vi "LabVIEW_INI_FIX_Fonts_2011.vi"() -> ()   [LabVIEW 2011]
uses:
  <vilib>/registry/registry.llb/Registry RtKey.ctl
  <vilib>/registry/registry.llb/Registry SAM.ctl
  <vilib>/Utility/config.llb/Read Key (String).vi
  <vilib>/Utility/config.llb/Write Key (String).vi
  <vilib>/Utility/config.llb/NI_LVConfig.lvlib
panel:
  out "total fonts info in registry":T1
  out "all fonts array":string[](array[string])
  out "Fonts sorted":string[](array[string])
  out "previous value in ini":string
  out "Fonts value to write in ini":string
  out "All found labVIEW.INI in Default Dir":path[](array[path])
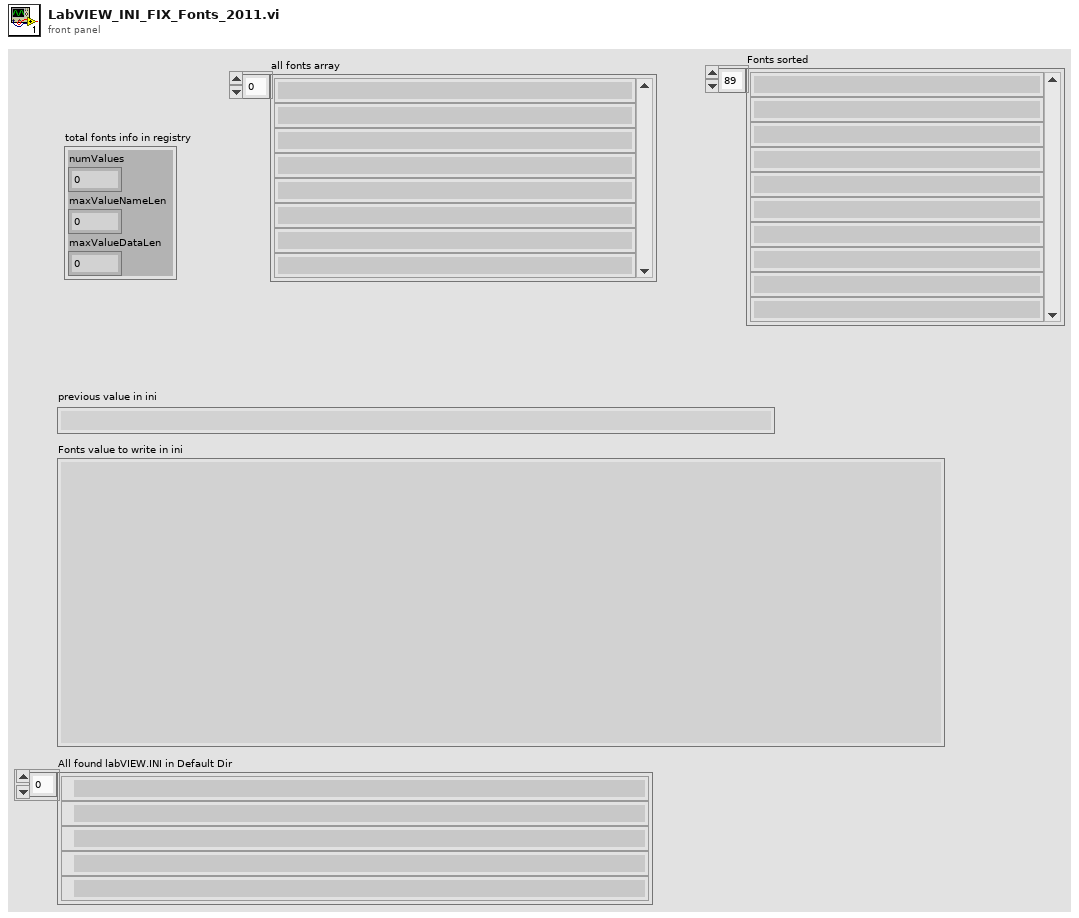
[diagram p1: front panel]
types:
  T1 = cluster{"numValues":i32, "maxValueNameLen":i32, "maxValueDataLen":i32}
  T2 = typedef "Registry SAM.ctl" = enum32{"KEY_QUERY_VALUE", "KEY_SET_VALUE", "KEY_CREATE_SUB_KEY", "KEY_ENUMERATE_SUB_KEYS", "KEY_NOTIFY", "KEY_CREATE_LINK", "KEY_READ", "KEY_WRITE", "KEY_ALL_ACCESS", "KEY_READ | KEY_WRITE"}
  T3 = typedef "Registry RtKey.ctl" = enum32{"HKEY_CLASSES_ROOT", "HKEY_CURRENT_USER", "HKEY_LOCAL_MACHINE", "HKEY_USERS", "HKEY_PERFORMANCE_DATA", "HKEY_CURRENT_CONFIG", "HKEY_DYN_DATA"}
  T4 = typedef "Registry refnum.ctl" = refnum<k1>
  T5 = typedef "NI_LVConfig.lvlib/Config Data RefNum.ctl" = refnum<k1>
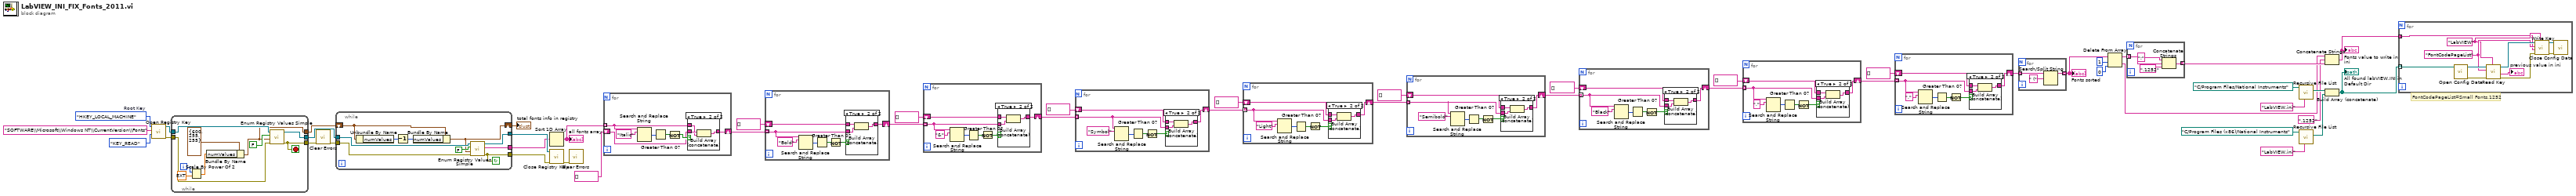
[diagram p0: block diagram]
diagram:
  w34 = Registry_RtKey."HKEY_LOCAL_MACHINE"  # Root Key
  # "FontCodePageList=Small Fonts,1252"
  n1 = call <vilib>:"Open Registry Key.vi"("security access mask (KEY_READ | KEY_WRITE)"=Registry_SAM."KEY_READ", "subkey"="SOFTWARE\\Microsoft\\Windows NT\\CurrentVersion\\Fonts", "root key (HKEY_LOCAL_MACHINE)"=w34) -> ("error out"=w15:errorcluster, "refnum out"=w18:T4)  [unwired: 7 in]
  n2 = while {
    tunnel: w18 -> [w57]
    tunnel: [w55] -> w19
    tunnel: [w51] -> w20
    tunnel: w15 -> [w50]
    tunnel: [w49] -> w14
    i -> [w54]
    stop <- w49 stop-if-true
    n3 = Scale By Power Of 2(n=w54, x=ext 1.0) -> (x*2^n=w52:ext)
    n4 = Bundle By Name(cluster=T1 {"numValues"=600, "maxValueNameLen"=255, "maxValueDataLen"=255} ("value info"), "numValues"=w52) -> (w51:T1)
    n5 = call <vilib>:"Enum Registry Values Simple.vi"("error in (no error)"=w50, "value info"=w51, "retrieve data? (F)"=FALSE, "refnum"=w57) -> ("error out"=w49:errorcluster, "refnum out"=w55:T4)  [unwired: 2 in, 4 out]
  }
  n6 = call <vilib>:"Clear Errors.vi"("error in (no error)"=w14) -> ("error out"=w12:errorcluster)  [unwired: 6 in]
  n7 = while {
    shift-right: [w62] -> w11
    shift-left: w20 -> [w67]
    tunnel: w19 -> [w64]
    tunnel: [w63] -> w17
    tunnel: [w61] -> w16
    tunnel: w12 -> [w60]
    tunnel: [w59] -> w13
    stop <- w59 continue-if-true
    n8 = Unbundle By Name(w67) -> ("numValues"=w66:i32)
    n9 = Decrement(x=w66) -> (x-1=w65:i32)
    n10 = Bundle By Name(cluster=w67, "numValues"=w65) -> (w62:T1)
    n11 = call <vilib>:"Enum Registry Values Simple.vi"("error in (no error)"=w60, "value info"=w62, "retrieve data? (F)"=FALSE, "refnum"=w64) -> ("error out"=w59:errorcluster, "values"=w61:string[], "refnum out"=w63:T4)  [unwired: 2 in, 3 out]
  }
  "total fonts info in registry" <- w11
  n12 = Sort 1D Array(array=w16) -> (sorted array=w26:string[])
  "all fonts array" <- w26
  n13 = call <vilib>:"Close Registry Key.vi"("error in (no error)"=w13, "refnum"=w17) -> ("error out"=w21:errorcluster)  [unwired: 5 in]
  n14 = call <vilib>:"Clear Errors.vi"("error in (no error)"=w21) -> ()  [unwired: 6 in, 1 out]
  n15 = for {
    tunnel: w26 -> [w72] mode=indexing
    shift-right: [w69] -> w31
    shift-left: string[] [] ("Array") -> [w70]
    n16 = Search and Replace String(input string=w72, search string="Italic") -> (number of replacements=w74:i32)  [unwired: 6 in, 3 out]
    n17 = Greater Than 0?(x=w74) -> (x > 0?=w73:bool)
    n18 = Not(x=w73) -> (.not. x?=w71:bool)
    n19 = case shown="True" w71 {
      tunnel: w70 -> [w76 w78]
      tunnel: w72 -> [_ w77]
      tunnel: [w76 w79] -> w69
      frame False {
      }
      frame True {
        n20 = Build Array (concatenate)(w78, w77) -> (w79:string[])
      }
    }
  }
  n21 = for {
    tunnel: w31 -> [w83] mode=indexing
    shift-right: [w80] -> w30
    shift-left: string[] [] ("Array") -> [w81]
    n22 = Search and Replace String(input string=w83, search string="Bold") -> (number of replacements=w85:i32)  [unwired: 6 in, 3 out]
    n23 = Greater Than 0?(x=w85) -> (x > 0?=w84:bool)
    n24 = Not(x=w84) -> (.not. x?=w82:bool)
    n25 = case shown="True" w82 {
      tunnel: w81 -> [w87 w89]
      tunnel: w83 -> [_ w88]
      tunnel: [w87 w90] -> w80
      frame False {
      }
      frame True {
        n26 = Build Array (concatenate)(w89, w88) -> (w90:string[])
      }
    }
  }
  n27 = for {
    tunnel: w30 -> [w94] mode=indexing
    shift-right: [w91] -> w29
    shift-left: string[] [] ("Array") -> [w92]
    n28 = Search and Replace String(input string=w94, search string="&") -> (number of replacements=w96:i32)  [unwired: 6 in, 3 out]
    n29 = Greater Than 0?(x=w96) -> (x > 0?=w95:bool)
    n30 = Not(x=w95) -> (.not. x?=w93:bool)
    n31 = case shown="True" w93 {
      tunnel: w92 -> [w98 w100]
      tunnel: w94 -> [_ w99]
      tunnel: [w98 w101] -> w91
      frame False {
      }
      frame True {
        n32 = Build Array (concatenate)(w100, w99) -> (w101:string[])
      }
    }
  }
  n33 = for {
    tunnel: w29 -> [w105] mode=indexing
    shift-right: [w102] -> w28
    shift-left: string[] [] ("Array") -> [w103]
    n34 = Search and Replace String(input string=w105, search string="Symbol") -> (number of replacements=w107:i32)  [unwired: 6 in, 3 out]
    n35 = Greater Than 0?(x=w107) -> (x > 0?=w106:bool)
    n36 = Not(x=w106) -> (.not. x?=w104:bool)
    n37 = case shown="True" w104 {
      tunnel: w103 -> [w109 w111]
      tunnel: w105 -> [_ w110]
      tunnel: [w109 w112] -> w102
      frame False {
      }
      frame True {
        n38 = Build Array (concatenate)(w111, w110) -> (w112:string[])
      }
    }
  }
  n39 = for {
    tunnel: w28 -> [w116] mode=indexing
    shift-right: [w113] -> w27
    shift-left: string[] [] ("Array") -> [w114]
    n40 = Search and Replace String(input string=w116, search string="Light") -> (number of replacements=w118:i32)  [unwired: 6 in, 3 out]
    n41 = Greater Than 0?(x=w118) -> (x > 0?=w117:bool)
    n42 = Not(x=w117) -> (.not. x?=w115:bool)
    n43 = case shown="True" w115 {
      tunnel: w114 -> [w120 w122]
      tunnel: w116 -> [_ w121]
      tunnel: [w120 w123] -> w113
      frame False {
      }
      frame True {
        n44 = Build Array (concatenate)(w122, w121) -> (w123:string[])
      }
    }
  }
  n45 = for {
    tunnel: w27 -> [w127] mode=indexing
    shift-right: [w124] -> w25
    shift-left: string[] [] ("Array") -> [w125]
    n46 = Search and Replace String(input string=w127, search string="Semibold") -> (number of replacements=w129:i32)  [unwired: 6 in, 3 out]
    n47 = Greater Than 0?(x=w129) -> (x > 0?=w128:bool)
    n48 = Not(x=w128) -> (.not. x?=w126:bool)
    n49 = case shown="True" w126 {
      tunnel: w125 -> [w131 w133]
      tunnel: w127 -> [_ w132]
      tunnel: [w131 w134] -> w124
      frame False {
      }
      frame True {
        n50 = Build Array (concatenate)(w133, w132) -> (w134:string[])
      }
    }
  }
  n51 = for {
    tunnel: w25 -> [w138] mode=indexing
    shift-right: [w135] -> w24
    shift-left: string[] [] ("Array") -> [w136]
    n52 = Search and Replace String(input string=w138, search string="Black") -> (number of replacements=w140:i32)  [unwired: 6 in, 3 out]
    n53 = Greater Than 0?(x=w140) -> (x > 0?=w139:bool)
    n54 = Not(x=w139) -> (.not. x?=w137:bool)
    n55 = case shown="True" w137 {
      tunnel: w136 -> [w142 w144]
      tunnel: w138 -> [_ w143]
      tunnel: [w142 w145] -> w135
      frame False {
      }
      frame True {
        n56 = Build Array (concatenate)(w144, w143) -> (w145:string[])
      }
    }
  }
  n57 = for {
    tunnel: w24 -> [w149] mode=indexing
    shift-right: [w146] -> w23
    shift-left: string[] [] ("Array") -> [w147]
    n58 = Search and Replace String(input string=w149, search string=",") -> (number of replacements=w151:i32)  [unwired: 6 in, 3 out]
    n59 = Greater Than 0?(x=w151) -> (x > 0?=w150:bool)
    n60 = Not(x=w150) -> (.not. x?=w148:bool)
    n61 = case shown="True" w148 {
      tunnel: w147 -> [w153 w155]
      tunnel: w149 -> [_ w154]
      tunnel: [w153 w156] -> w146
      frame False {
      }
      frame True {
        n62 = Build Array (concatenate)(w155, w154) -> (w156:string[])
      }
    }
  }
  n63 = for {
    tunnel: w23 -> [w160] mode=indexing
    shift-right: [w157] -> w22
    shift-left: string[] [] ("Array") -> [w158]
    n64 = Search and Replace String(input string=w160, search string=",") -> (number of replacements=w162:i32)  [unwired: 6 in, 3 out]
    n65 = Greater Than 0?(x=w162) -> (x > 0?=w161:bool)
    n66 = Not(x=w161) -> (.not. x?=w159:bool)
    n67 = case shown="True" w159 {
      tunnel: w158 -> [w164 w166]
      tunnel: w160 -> [_ w165]
      tunnel: [w164 w167] -> w157
      frame False {
      }
      frame True {
        n68 = Build Array (concatenate)(w166, w165) -> (w167:string[])
      }
    }
  }
  n69 = for {
    tunnel: w22 -> [w170] mode=indexing
    tunnel: [w168] -> w1 mode=indexing
    n70 = Search/Split String(string=w170, search string/char (-)=" (") -> (substring before match=w168:string)  [unwired: 1 in, 2 out]
  }
  "Fonts sorted" <- w1
  n71 = Delete From Array(array=w1, length=1, index=0) -> (deleted portion=w36:string[], array with subset deleted=w40:string[])
  n72 = for {
    tunnel: w40 -> [w174] mode=indexing
    tunnel: [w172] -> w41 mode=indexing
    n73 = Concatenate Strings(";" ("string"), w174, ",1252" ("string")) -> (w172:string)
  }
  n74 = call <vilib>:"Recursive File List.vi"("pattern"="LabVIEW.ini", "Folder Path"=path "C:/Program Files/National Instruments") -> ("All Files in Dir"=w44:path[])  [unwired: 5 in, 4 out]
  n75 = call <vilib>:"Recursive File List.vi"("pattern"="LabVIEW.ini", "Folder Path"=path "C:/Program Files (x86)/National Instruments") -> ("All Files in Dir"=w43:path[])  [unwired: 5 in, 4 out]
  n76 = Concatenate Strings(w36, ",1252" ("string"), w41) -> (w35:string)
  "Fonts value to write in ini" <- w35
  n77 = Build Array (concatenate)(w44, w43) -> (w42:path[])
  "All found labVIEW.INI in Default Dir" <- w42
  n78 = for {
    tunnel: w42 -> [w179] mode=indexing
    tunnel: w35 -> [w175]
    w177 = "FontCodePageList" ("key")
    w176 = "LabVIEW" ("section")
    n79 = call <vilib>:"Open Config Data.vi"("configuration file path"=w179) -> ("error out"=w183:errorcluster, "refnum"=w182:T5)  [unwired: 8 in, 1 out]
    n80 = call-poly <vilib>:"Read Key.vi"("section"=w176, "error in (no error)"=w183, "key"=w177, "refnum"=w182) -> ("error out"=w180:errorcluster, "value"=→"previous value in ini":string, "refnum out"=w181:T5)  [unwired: 4 in, 1 out]
    n81 = call-poly <vilib>:"Write Key.vi"("section"=w176, "error in (no error)"=w180, "value"=w175, "key"=w177, "refnum"=w181) -> ("error out"=w185:errorcluster, "refnum out"=w184:T5)  [unwired: 4 in, 1 out]
    n82 = call <vilib>:"Close Config Data.vi"("error in (no error)"=w185, "refnum"=w184) -> ()  [unwired: 8 in, 2 out]
  }
